vi "1TwoSum.vi"(8 "error in (no error)":errorcluster, 10 "Target":i32, 11 "Nums":i32[](array[numeric])) -> (0 "error out":errorcluster, 3 "Output":i32[](array[numeric]))   [LabVIEW 2023]
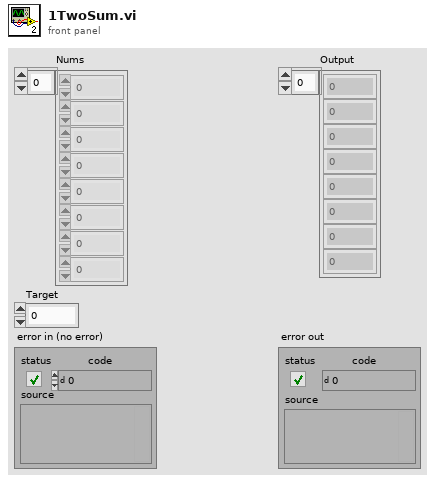
[diagram p1: front panel]
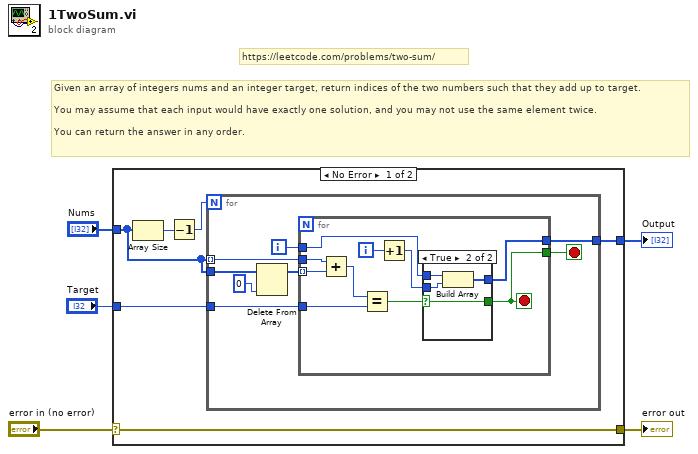
[diagram p0: block diagram]
diagram:
  # "Given an array of integers nums and an integer target, return indices of the two numbers such that they add up to target.\n\nYou may assume that each input would have exactly one solution, and you may not use the same element twice.\n\nYou can return the answer in any order."
  # "https://leetcode.com/problems/two-sum/"
  n1 = case shown="No Error" "error in (no error)" {
    selector: "error in (no error)" -> [w10 w35]
    tunnel: "Target" -> [w11 _]
    tunnel: "Nums" -> [w8 _]
    tunnel: [w10 w35] -> w2
    tunnel: [w6 _] -> w1
    frame No Error {
      n2 = Array Size(array=w8) -> (size(s)=w9:i32)
      n3 = Decrement(x=w9) -> (x-1=w7:i32)
      n4 = for {
        N: w7 -> [_]
        tunnel: w11 -> [w17]
        tunnel: w8 -> [w19] mode=indexing
        tunnel: w8 -> [w18]
        tunnel: [w14] -> w6
        i -> [w16]
        stop <- w12 stop-if-true
        n5 = Delete From Array(array=w18, index=0) -> (array with subset deleted=w15:i32[])  [unwired: 1 in, 1 out]
        n6 = for {
          tunnel: w19 -> [w29]
          tunnel: w15 -> [w28] mode=indexing
          tunnel: w17 -> [w27]
          tunnel: w16 -> [w24]
          tunnel: [w22] -> w14
          tunnel: [w21] -> w12
          i -> [w23]
          stop <- w21 stop-if-true
          n7 = Add(x=w29, y=w28) -> (x+y=w26:i32)
          n8 = Equal?(x=w26, y=w27) -> (x = y?=w25:bool)
          n9 = Increment(x=w23) -> (x+1=w20:i32)
          n10 = case shown="True" w25 {
            selector: w25 -> [w30 w31]
            tunnel: w24 -> [_ w34]
            tunnel: w20 -> [_ w33]
            tunnel: [_ w32] -> w22
            tunnel: [w30 w31] -> w21
            frame False {
            }
            frame True {
              n11 = Build Array(w34, w33) -> (w32:i32[])
            }
          }
        }
      }
    }
    frame Error {
    }
  }
  "Output" <- w1
  "error out" <- w2
